vi "Application.vi"() -> ()   [LabVIEW 2020]
panel:
  out "Bottom Box?":bool
  out "Top box?":bool
  out "Image":T1(plugin-control)
  out "Top plate?":bool
  out "White side?":bool
  out "White side hole?":bool
  in  "Match":bool
  in  "Stop Button":bool
  in  "Image File Path":path
  in  "Read Next Image":bool
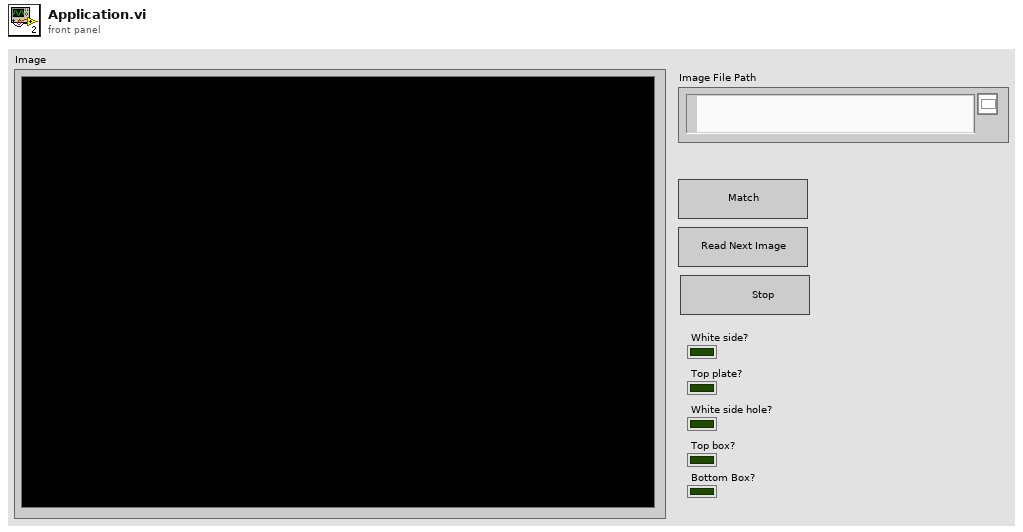
[diagram p1: front panel]
types:
  T1 = typedef "IMAQ Image.ctl" = refnum<image>
  T2 = typedef "Image Type" = u32
  T3 = cluster{"Position":cluster{"x":sgl, "y":sgl}, "Angle":sgl, "Scale":sgl, "Score":sgl, "Bounding Box":cluster{"x":sgl, "y":sgl}[]}[]
  T4 = cluster{"Position":cluster{"x":sgl, "y":sgl}, "Angle":sgl, "Scale":sgl, "Score":sgl, "Bounding Box":cluster{"x":sgl, "y":sgl}[]}[][]
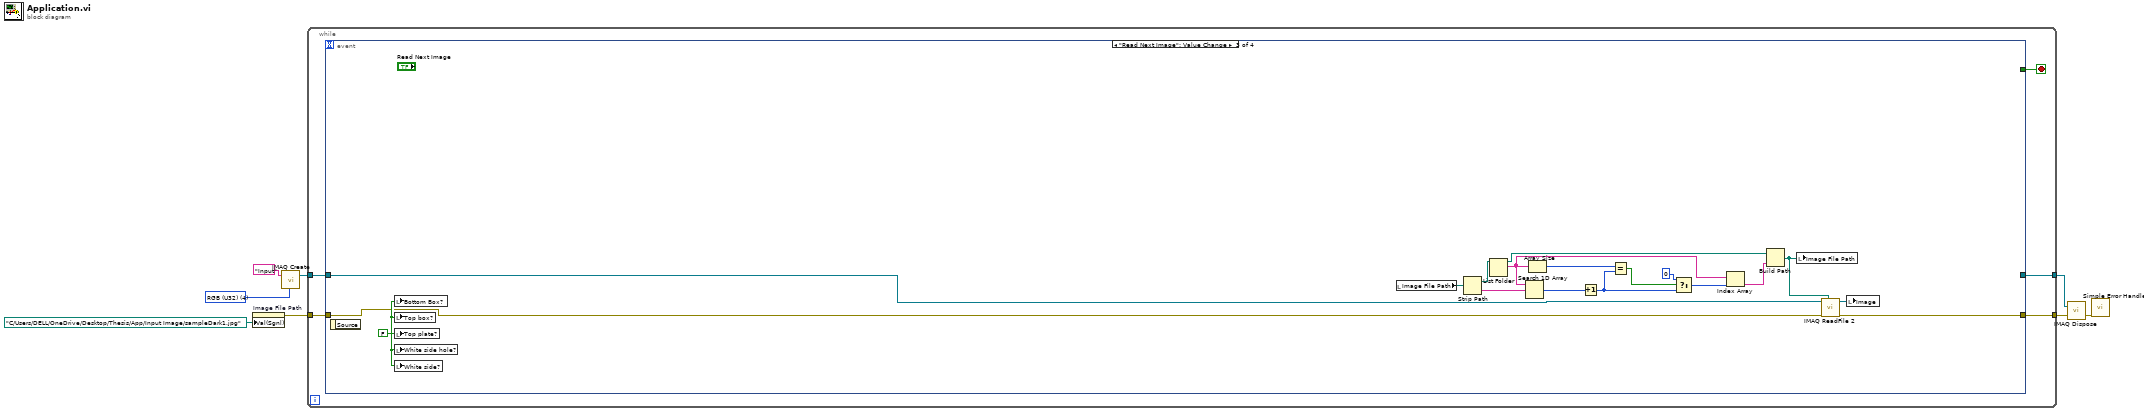
[diagram p0: block diagram]
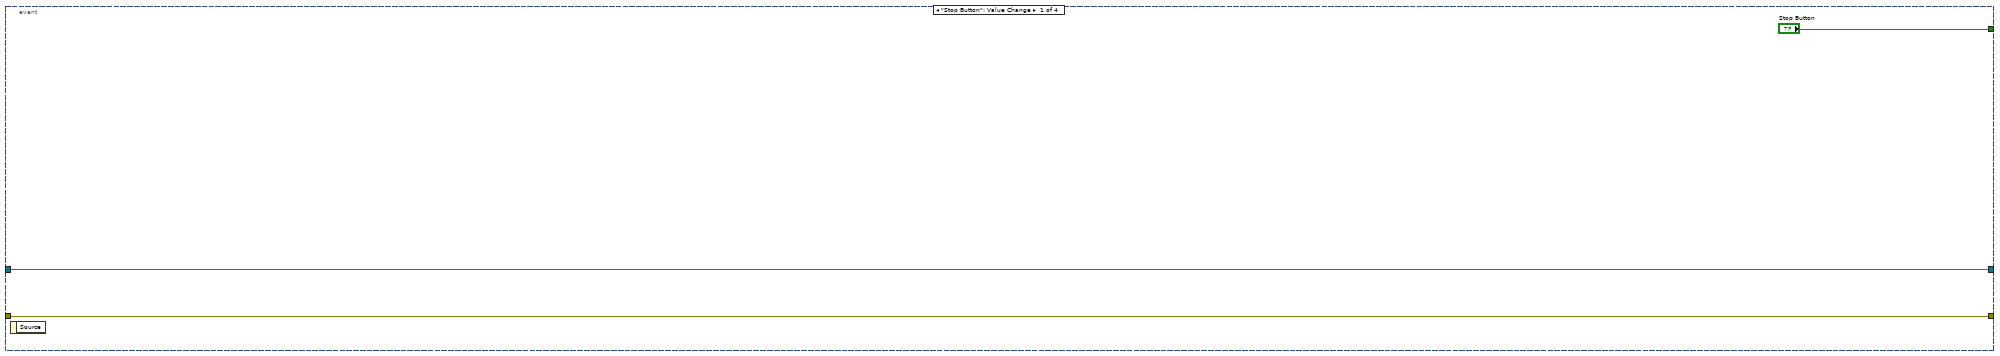
[diagram p2: hidden frame]
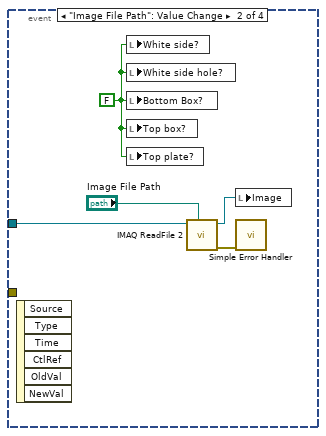
[diagram p3: hidden frame]
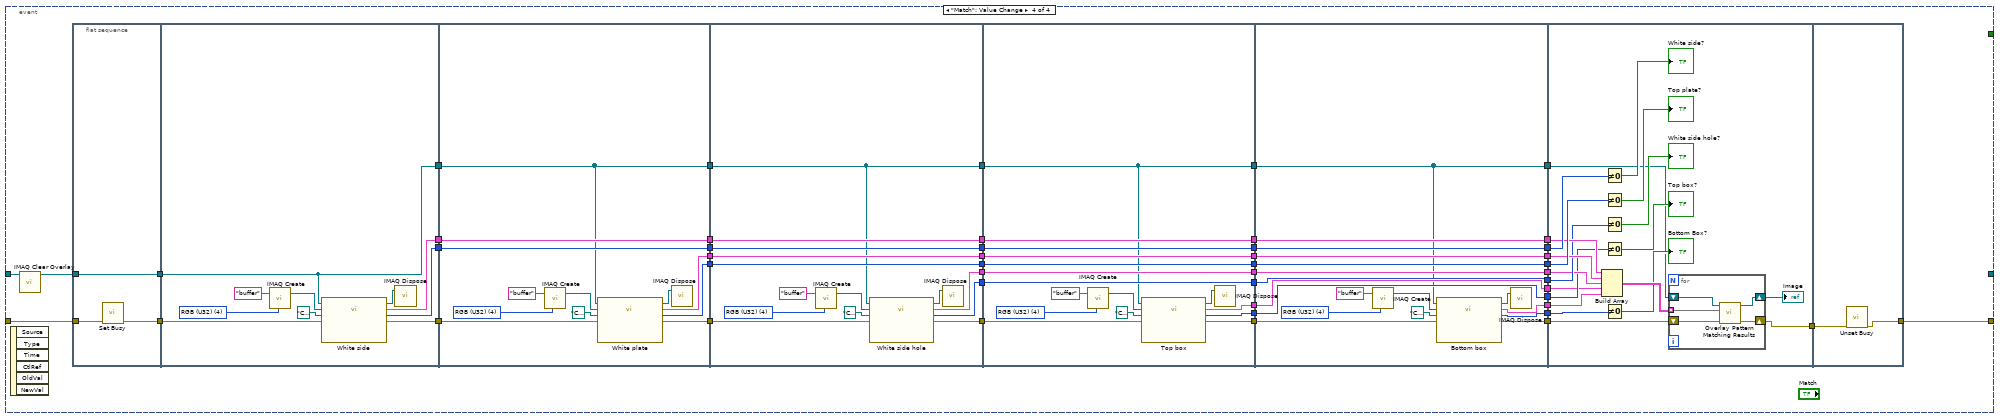
[diagram p4: hidden frame]
diagram:
  w5 = T2 4 items=["Grayscale (U8)", "Grayscale (I16)", "Grayscale (SGL)", "Complex (CSG)", "RGB (U32)", "HSL (U32)", "RGB (U64)", "Grayscale (U16)"] ("Image Type")
  n1 = property on="Image File Path" class="Path"("Val(Sgnl)"=path "C:/Users/DELL/OneDrive/Desktop/Thesis/App/Input Image/sampleDark1.jpg" ("Value (Signaling)")) -> (error out=w2:errorcluster)  [unwired: 2 in, 1 out]
  n2 = call "IMAQ Create"("Image Name"="Input", "Image Type"=w5) -> ("New Image"=w4:T1)  [unwired: 3 in, 1 out]
  n3 = while {
    tunnel: w4 -> [w12]
    tunnel: w2 -> [w11]
    tunnel: [w10] -> w7
    tunnel: [w9] -> w6
    stop <- w13 stop-if-true
    n4 = event shown="[2] \"Read Next Image\": Value Change" {
      selector: _ -> [_ _ _ _]
      dyn-events: _ -> [_ _ _ _]
      timeout: _ -> [_ _ _ _]
      tunnel: ["Stop Button" _ _ _] -> w13
      tunnel: w12 -> [w16 w21 w25 w86]
      tunnel: w11 -> [w14 _ w22 w83]
      tunnel: [w16 _ _ _] -> w10
      tunnel: [w14 _ w24 w40] -> w9
      event "Stop Button": Value Change {
        n5 = event-data() -> ()  [unwired: 1 in, 1 out]
      }
      event "Image File Path": Value Change {
        w17 = FALSE
        n6 = event-data() -> ()  [unwired: 1 in, 6 out]
        n7 = local write "White side?"(w17) -> ()
        n8 = local write "White side hole?"(w17) -> ()
        n9 = local write "Bottom Box?"(w17) -> ()
        n10 = local write "Top box?"(w17) -> ()
        n11 = local write "Top plate?"(w17) -> ()
        n12 = call "IMAQ ReadFile 2"("File Path"="Image File Path", "Image"=w21) -> ("error out"=w18:errorcluster, "Image Out"=w20:T1)  [unwired: 5 in, 3 out]
        n13 = local write "Image"(w20) -> ()
        n14 = call <vilib>:"Simple Error Handler.vi"("error in (no error)"=w18) -> ()  [unwired: 4 in, 5 out]
      }
      event "Read Next Image": Value Change {
        w23 = FALSE
        n15 = event-data() -> ()  [unwired: 1 in, 1 out]
        n16 = local write "Bottom Box?"(w23) -> ()
        n17 = local write "Top box?"(w23) -> ()
        n18 = local write "Top plate?"(w23) -> ()
        n19 = local write "White side hole?"(w23) -> ()
        n20 = local write "White side?"(w23) -> ()
        n21 = local read "Image File Path"() -> (w28:path)
        n22 = Strip Path(path=w28) -> (stripped path=w29:path, name=w30:string)
        n23 = List Folder(path=w29) -> (path out=w34:path, filenames=w32:string[])  [unwired: 3 in, 2 out]
        n24 = Search 1D Array(1D array=w32, element=w30) -> (index of element=w31:i32)  [unwired: 1 in]
        n25 = Array Size(array=w32) -> (size(s)=w36:i32)
        n26 = Increment(x=w31) -> (x+1=w39:i32)
        n27 = Equal?(x=w36, y=w39) -> (x = y?=w37:bool)
        n28 = Select(t=0 ("x+1"), s=w37, f=w39) -> (s? t:f=w38:i32)
        n29 = Index Array(array=w32, index=w38) -> (element=w33:string)
        n30 = Build Path(base path=w34, name or relative path=w33) -> (appended path=w35:path)
        n31 = local write "Image File Path"(w35) -> ()
        n32 = call "IMAQ ReadFile 2"("File Path"=w35, "error in (no error)"=w22, "Image"=w25) -> ("error out"=w24:errorcluster, "Image Out"=w27:T1)  [unwired: 4 in, 3 out]
        n33 = local write "Image"(w27) -> ()
      }
      event "Match": Value Change {
        n34 = event-data() -> ()  [unwired: 1 in, 6 out]
        n35 = call "IMAQ Clear Overlay"("Image"=w86) -> ("Image Out"=w85:T1)  [unwired: 9 in, 1 out]
        n36 = flat-sequence {
          tunnel: w83 -> [w88]
          tunnel: w85 -> [w89]
          tunnel: [w89] -> w43
          tunnel: [w87] -> w42
          tunnel: [w94] -> w84
          tunnel: [w97] -> w78
          tunnel: [w98] -> w77
          tunnel: [w96] -> w76
          tunnel: w43 -> [w94]
          tunnel: w42 -> [w99]
          tunnel: w84 -> [w104]
          tunnel: [w111] -> w79
          tunnel: w78 -> [w111]
          tunnel: w77 -> [w109]
          tunnel: w76 -> [w105]
          tunnel: [w108] -> w72
          tunnel: [w107] -> w71
          tunnel: [w106] -> w70
          tunnel: [w105] -> w66
          tunnel: [w104] -> w47
          tunnel: [w125] -> w80
          tunnel: w79 -> [w125]
          tunnel: [w124] -> w73
          tunnel: w72 -> [w124]
          tunnel: w71 -> [w120]
          tunnel: w70 -> [w122]
          tunnel: [w123] -> w67
          tunnel: w66 -> [w123]
          tunnel: [w122] -> w63
          tunnel: [w119] -> w60
          tunnel: [w118] -> w59
          tunnel: [w117] -> w56
          tunnel: w47 -> [w116]
          tunnel: [w116] -> w46
          tunnel: [w141] -> w81
          tunnel: w80 -> [w141]
          tunnel: [w140] -> w74
          tunnel: w73 -> [w140]
          tunnel: [w139] -> w68
          tunnel: w67 -> [w139]
          tunnel: [w138] -> w64
          tunnel: w63 -> [w138]
          tunnel: [w137] -> w61
          tunnel: w60 -> [w137]
          tunnel: w59 -> [w134]
          tunnel: [w136] -> w57
          tunnel: w56 -> [w136]
          tunnel: [w133] -> w55
          tunnel: [w132] -> w53
          tunnel: [w131] -> w51
          tunnel: w46 -> [w130]
          tunnel: [w130] -> w45
          tunnel: [w159] -> w82
          tunnel: w81 -> [w159]
          tunnel: [w158] -> w75
          tunnel: w74 -> [w158]
          tunnel: [w157] -> w69
          tunnel: w68 -> [w157]
          tunnel: [w156] -> w65
          tunnel: w64 -> [w156]
          tunnel: [w155] -> w62
          tunnel: w61 -> [w155]
          tunnel: [w154] -> w58
          tunnel: w57 -> [w154]
          tunnel: w55 -> [w150]
          tunnel: [w153] -> w54
          tunnel: w53 -> [w153]
          tunnel: [w152] -> w52
          tunnel: w51 -> [w152]
          tunnel: [w149] -> w50
          tunnel: [w148] -> w49
          tunnel: [w147] -> w48
          tunnel: w45 -> [w146]
          tunnel: [w146] -> w44
          tunnel: w82 -> [w178]
          tunnel: w75 -> [w176]
          tunnel: w69 -> [w173]
          tunnel: w65 -> [w172]
          tunnel: w62 -> [w170]
          tunnel: w58 -> [w169]
          tunnel: w54 -> [w167]
          tunnel: w52 -> [w166]
          tunnel: w50 -> [w164]
          tunnel: w49 -> [w163]
          tunnel: w48 -> [w162]
          tunnel: w44 -> [w161]
          tunnel: [w160] -> w41
          tunnel: w41 -> [w186]
          tunnel: [w185] -> w40
          frame #0 {
            n37 = call <vilib>:"Set Busy.vi"("error in (no error)"=w88) -> ("error out"=w87:errorcluster)  [unwired: 9 in, 1 out]
          }
          frame #1 {
            w92 = T2 4 items=["Grayscale (U8)", "Grayscale (I16)", "Grayscale (SGL)", "Complex (CSG)", "RGB (U32)", "HSL (U32)", "RGB (U64)", "Grayscale (U16)"] ("Image Type")
            n38 = call "IMAQ Create"("Image Name"="buffer", "Image Type"=w92) -> ("New Image"=w91:T1)  [unwired: 3 in, 1 out]
            n39 = call "White side"("Image In"=w94, "Image Dst"=w91, "Template File Path (Pattern Matching 1)"=path "C:/Users/DELL/OneDrive/Desktop/Thesis/App/Matching template/plateSideTemplate.png", "error in"=w99) -> ("Image Out"=w90:T1, "Matches (Pattern Matching 1)"=w96:T3, "Number of Matches (Pattern Matching 1)"=w97:i32, "error out"=w98:errorcluster)  [unwired: 20 in]
            n40 = call "IMAQ Dispose"("Image"=w90) -> ()  [unwired: 5 in, 1 out]
          }
          frame #2 {
            w102 = T2 4 items=["Grayscale (U8)", "Grayscale (I16)", "Grayscale (SGL)", "Complex (CSG)", "RGB (U32)", "HSL (U32)", "RGB (U64)", "Grayscale (U16)"] ("Image Type")
            n41 = call "IMAQ Create"("Image Name"="buffer", "Image Type"=w102) -> ("New Image"=w101:T1)  [unwired: 3 in, 1 out]
            n42 = call "White plate"("Image In"=w104, "Image Dst"=w101, "Template File Path (Pattern Matching 1)"=path "C:/Users/DELL/OneDrive/Desktop/Thesis/App/Matching template/plateTopTemplate.png", "error in"=w109) -> ("Image Out"=w100:T1, "Matches (Pattern Matching 1)"=w106:T3, "Number of Matches (Pattern Matching 1)"=w108:i32, "error out"=w107:errorcluster)  [unwired: 20 in]
            n43 = call "IMAQ Dispose"("Image"=w100) -> ()  [unwired: 5 in, 1 out]
          }
          frame #3 {
            w114 = T2 4 items=["Grayscale (U8)", "Grayscale (I16)", "Grayscale (SGL)", "Complex (CSG)", "RGB (U32)", "HSL (U32)", "RGB (U64)", "Grayscale (U16)"] ("Image Type")
            n44 = call "IMAQ Create"("Image Name"="buffer", "Image Type"=w114) -> ("New Image"=w113:T1)  [unwired: 3 in, 1 out]
            n45 = call "White side hole"("Image In"=w116, "Image Dst"=w113, "Template File Path (Pattern Matching 1)"=path "C:/Users/DELL/OneDrive/Desktop/Thesis/App/Matching template/plateSideHoldTemplate.png", "error in"=w120) -> ("Image Out"=w112:T1, "Matches (Pattern Matching 1)"=w117:T3, "Number of Matches (Pattern Matching 1)"=w119:i32, "error out"=w118:errorcluster)  [unwired: 20 in]
            n46 = call "IMAQ Dispose"("Image"=w112) -> ()  [unwired: 5 in, 1 out]
          }
          frame #4 {
            w128 = T2 4 items=["Grayscale (U8)", "Grayscale (I16)", "Grayscale (SGL)", "Complex (CSG)", "RGB (U32)", "HSL (U32)", "RGB (U64)", "Grayscale (U16)"] ("Image Type")
            n47 = call "IMAQ Create"("Image Name"="buffer", "Image Type"=w128) -> ("New Image"=w127:T1)  [unwired: 3 in, 1 out]
            n48 = call "Top box"("Image In"=w130, "Image Dst"=w127, "Template File Path (Pattern Matching 2)"=path "C:/Users/DELL/OneDrive/Desktop/Thesis/App/Matching template/boxTopTemplateSaturation.png", "error in"=w134) -> ("Image Out"=w126:T1, "Matches (Pattern Matching 2)"=w131:T3, "Number of Matches (Pattern Matching 2)"=w132:i32, "error out"=w133:errorcluster)  [unwired: 20 in]
            n49 = call "IMAQ Dispose"("Image"=w126) -> ()  [unwired: 5 in, 1 out]
          }
          frame #5 {
            w144 = T2 4 items=["Grayscale (U8)", "Grayscale (I16)", "Grayscale (SGL)", "Complex (CSG)", "RGB (U32)", "HSL (U32)", "RGB (U64)", "Grayscale (U16)"] ("Image Type")
            n50 = call "IMAQ Create"("Image Name"="buffer", "Image Type"=w144) -> ("New Image"=w143:T1)  [unwired: 3 in, 1 out]
            n51 = call "Bottom box"("Image In"=w146, "Image Dst"=w143, "Template File Path (Pattern Matching 2)"=path "C:/Users/DELL/OneDrive/Desktop/Thesis/App/Matching template/boxBottomTemplateSaturation.png", "error in"=w150) -> ("Image Out"=w142:T1, "Matches (Pattern Matching 2)"=w147:T3, "Number of Matches (Pattern Matching 2)"=w149:i32, "error out"=w148:errorcluster)  [unwired: 20 in]
            n52 = call "IMAQ Dispose"("Image"=w142) -> ()  [unwired: 5 in, 1 out]
          }
          frame #6 {
            n53 = Build Array(w173, w172, w169, w166, w162) -> (w175:T4)
            n54 = Not Equal To 0?(x=w178) -> (x != 0?=→"White side?":bool)
            n55 = Not Equal To 0?(x=w176) -> (x != 0?=→"Top plate?":bool)
            n56 = Not Equal To 0?(x=w170) -> (x != 0?=→"White side hole?":bool)
            n57 = Not Equal To 0?(x=w167) -> (x != 0?=→"Top box?":bool)
            n58 = Not Equal To 0?(x=w164) -> (x != 0?=→"Bottom Box?":bool)
            n59 = for {
              tunnel: w175 -> [w184] mode=indexing
              shift-right: [w183] -> w174
              shift-left: w161 -> [w182]
              shift-right: [w181] -> w160
              shift-left: w163 -> [w180]
              n60 = call "Overlay Pattern Matching Results.vi"("error in"=w180, "Matches"=w184, "Image"=w182) -> ("error out"=w181:errorcluster, "Image Out"=w183:T1)  [unwired: 7 in]
            }
            "Image" <- w174
          }
          frame #7 {
            n61 = call <vilib>:"Unset Busy.vi"("error in (no error)"=w186) -> ("error out"=w185:errorcluster)  [unwired: 10 in]
          }
        }
      }
    }
  }
  n62 = call "IMAQ Dispose"("Image"=w7, "error in (no error)"=w6) -> ("error out"=w1:errorcluster)  [unwired: 4 in]
  n63 = call <vilib>:"Simple Error Handler.vi"("error in (no error)"=w1) -> ()  [unwired: 4 in, 5 out]
